vi "Set Up Front Panel.vi"(8 "Error In":errorcluster) -> (0 "Error Out":errorcluster, 1 "Dual Mode Thermometer Indicator":refnum<class "Dual Mode Thermometer.lvclass">, 2 "Dual Mode Thermometer Control":refnum<class "Dual Mode Thermometer.lvclass">)   [LabVIEW 2014]
doc: "Creates and shows the \"front panel\", and also returns references to the Thermometer controls and indicators.\n\n\nCopyright (c) 2019 Sze Howe Koh.\nThis code is licensed under the MIT license."
uses:
  Dual Mode Thermometer/Dual Mode Thermometer.lvclass
  <vilib>/addons/LQ/Qt Widgets/QBoxLayout/Direction.ctl
  Dual Mode Thermometer/Set Read Only.vi
  <vilib>/addons/LQ/Qt Widgets/QWidget/setVisible.vi
  <vilib>/addons/LQ/Qt Widgets/QWidget/QWidget.lvclass
  <vilib>/addons/LQ/Qt Widgets/QBoxLayout/QBoxLayout.lvclass
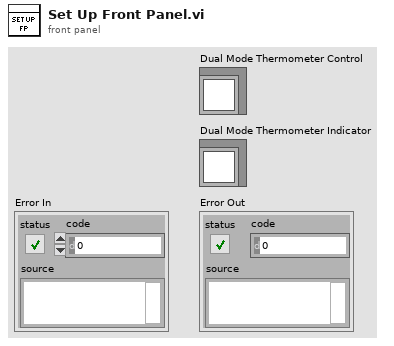
[diagram p1: front panel]
types:
  T1 = typedef "QBoxLayout.lvclass/Direction.ctl" = i32
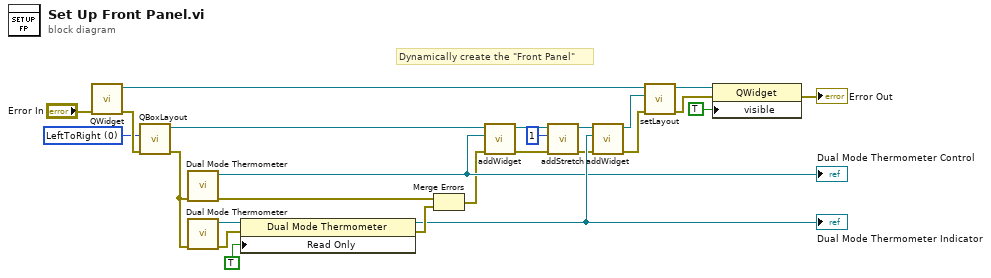
[diagram p0: block diagram]
diagram:
  w1 = T1 0 items=["LeftToRight", "RightToLeft", "TopToBottom", "BottomToTop"] ("direction")
  # "Dynamically create the \"Front Panel\""
  n1 = call <vilib>:"QWidget.vi"("Error In"="Error In") -> ("Error Out"=w16:errorcluster, "New QWidget"=w4:refnum<class "QWidget.lvclass">)  [unwired: 9 in]
  n2 = call <vilib>:"QBoxLayout.vi"("Error In"=w16, "direction"=w1) -> ("Error Out"=w17:errorcluster, "New QBoxLayout"=w7:refnum<class "QBoxLayout.lvclass">)  [unwired: 8 in]
  n3 = call "Dual Mode Thermometer.vi"("Error In"=w17) -> ("Error Out"=w18:errorcluster, "New Dual Mode Thermometer"=w13:refnum<class "Dual Mode Thermometer.lvclass">)  [unwired: 9 in]
  "Dual Mode Thermometer Control" <- w13
  n4 = call "Dual Mode Thermometer.vi"("Error In"=w17) -> ("Error Out"=w2:errorcluster, "New Dual Mode Thermometer"=w19:refnum<class "Dual Mode Thermometer.lvclass">)  [unwired: 9 in]
  n5 = property class="Dual Mode Thermometer"(reference=w19, error in=w2, "Read Only"=TRUE) -> (reference out=w24:refnum<class "Dual Mode Thermometer.lvclass">, error out=w25:errorcluster)
  "Dual Mode Thermometer Indicator" <- w24
  n6 = Merge Errors(w18, w25) -> (w3:errorcluster)
  n7 = call <vilib>:"addWidget.vi"("Error In"=w3, "widget"=w13, "QBoxLayout In"=w7) -> ("Error Out"=w10:errorcluster, "QBoxLayout Out"=w8:refnum<class "QBoxLayout.lvclass">)  [unwired: 7 in]
  n8 = call <vilib>:"addStretch.vi"("Error In"=w10, "stretch"=1, "QBoxLayout In"=w8) -> ("Error Out"=w12:errorcluster, "QBoxLayout Out"=w11:refnum<class "QBoxLayout.lvclass">)  [unwired: 7 in]
  n9 = call <vilib>:"addWidget.vi"("Error In"=w12, "widget"=w24, "QBoxLayout In"=w11) -> ("Error Out"=w20:errorcluster, "QBoxLayout Out"=w14:refnum<class "QBoxLayout.lvclass">)  [unwired: 7 in]
  n10 = call <vilib>:"setLayout.vi"("Error In"=w20, "layout"=w14, "QWidget In"=w4) -> ("Error Out"=w21:errorcluster, "QWidget Out"=w6:refnum<class "QWidget.lvclass">)  [unwired: 7 in]
  n11 = property class="QWidget"(reference=w6, error in=w21, "visible"=TRUE) -> (error out=→"Error Out":errorcluster)  [unwired: 1 out]
